vi "Read Device Load Statusvi.vi"(11 "Start Device Status Msg in":refnum<class "Device Load Status Msg.lvclass">) -> (0 "Status":T1, 1 "IED Name":string, 2 "CID Filename":string, 3 "Start Device Status Msg out":refnum<class "Device Load Status Msg.lvclass">, 4 "Error String":string)   [LabVIEW 2015, in "SCADA Core.lvlib" / "Device Load Status Msg.lvclass"]
uses:
  Device Load Status Msg.lvclass
  Device Load Status.ctl
  Device Load Status Msg.lvclass/Device Load Status Msg.ctl
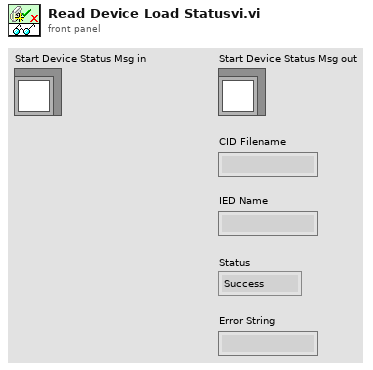
[diagram p1: front panel]
types:
  T1 = typedef "SCADA Core.lvlib/Device Load Status Msg.lvclass/Device Load Status.ctl" = enum16{"Success", "Failure"}
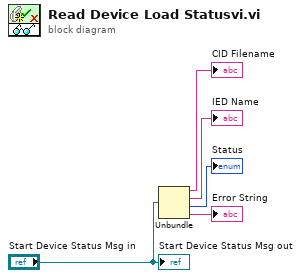
[diagram p0: block diagram]
diagram:
  n1 = Unbundle("Start Device Status Msg in") -> (→"CID Filename":string, →"IED Name":string, →"Status":T1, →"Error String":string)
  "Start Device Status Msg out" <- "Start Device Status Msg in"
